vi "SharedVar-subscriber.vi"() -> ()   [LabVIEW 2020]
uses:
  <vilib>/measure/maspectr.llb/FFT Power Spectrum and PSD for 1 Chan.vi
  <vilib>/measure/NI_MAPro.lvlib
panel:
  in  "stop":bool
  in  "Logarithmic Scale":bool
  in  "Window":u32(ring)=1 items=["Rectangle"=0, "Hanning"=1, "Hamming"=2, "Blackman-Harris"=3, "Exact Blackman"=4, "Blackman"=5, "Flat Top"=6, "4 Term B-Harris "=7, "7 Term B-Harris"=8, "Low Sidelobe"=9, "Blackman Nuttall"=11, "Triangle"=30, "Bartlett-Hanning"=31, "Bohman"=32, "Parzen"=33, "Welch"=34, "Kaiser"=60, "Dolph-Chebyshev"=61, "Gaussian"=62]
  out "Signal Waveform":waveform(dbl)(graph)
  out "Frequency Spectrum":cluster{"f0":dbl, "df":dbl, "magnitude":dbl[]}(graph)
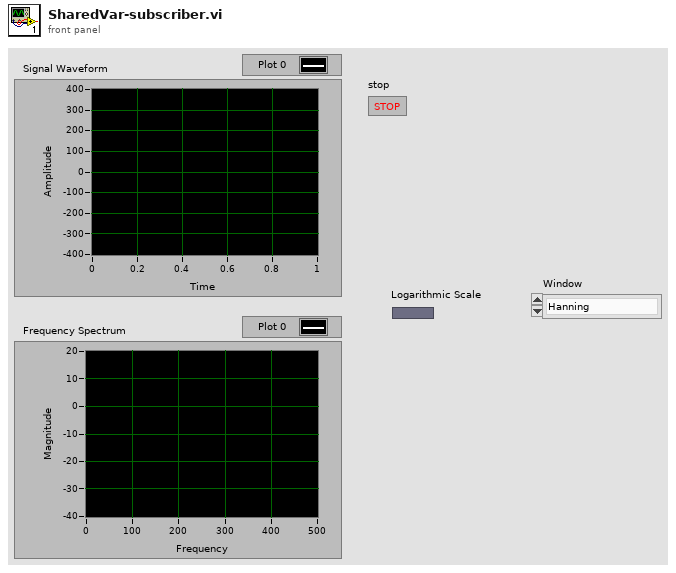
[diagram p1: front panel]
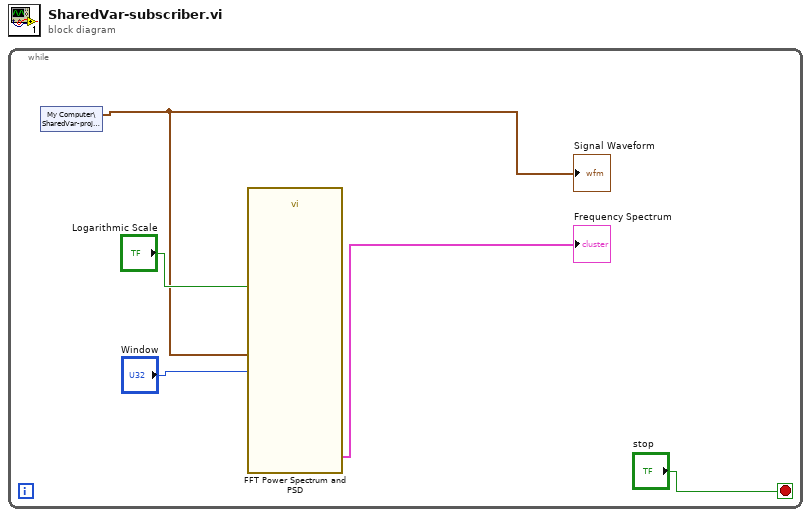
[diagram p0: block diagram]
diagram:
  n1 = while {
    stop <- "stop" stop-if-true
    n2 = shared-variable "My Computer\\SharedVar-project.lvlib\\Var"() -> (w2:waveform(dbl))  [unwired: 1 in, 1 out]
    "Signal Waveform" <- w2
    n3 = call-poly <vilib>:"FFT Power Spectrum and PSD.vi"("dB On (F)"="Logarithmic Scale", "window"="Window", "time signal"=w2) -> ("Power Spectrum / PSD"=→"Frequency Spectrum":cluster{"f0":dbl, "df":dbl, "magnitude":dbl[]})  [unwired: 5 in, 3 out]
  }
